vi "Mouse Down Signal.vi"(8 "error in (no error)":errorcluster, 11 "Handle in":refnum<class "Handle.lvclass">) -> (0 "error out":errorcluster, 3 "Handle out":refnum<class "Handle.lvclass">)   [LabVIEW 2021, in "Autocomplete Textbox.lvlib" / "Handle.lvclass"]
uses:
  Handle.lvclass
  ToMain UE.ctl
  ToMain UE action.ctl
  Handle.lvclass/Handle.ctl
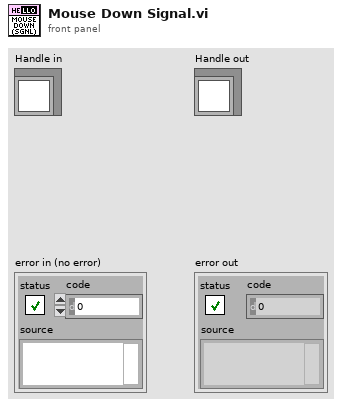
[diagram p1: front panel]
types:
  T1 = typedef "Autocomplete Textbox.lvlib/Handle.lvclass/ToMain UE action.ctl" = enum16{"New List", "Shutdown", "New Value", "Mouse Down (signal)"}
  T2 = typedef "Autocomplete Textbox.lvlib/Handle.lvclass/ToMain UE.ctl" = cluster{"Type":T1, "data":variant}
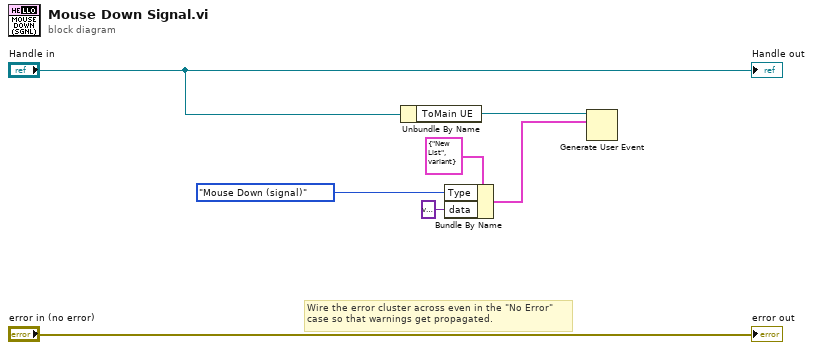
[diagram p0: block diagram]
diagram:
  # "Wire the error cluster across even in the \"No Error\"\ncase so that warnings get propagated."
  n1 = Unbundle By Name("Handle in") -> ("ToMain UE"=w6:refnum<user-event>)
  n2 = Bundle By Name(cluster=T2 {"Type"=enum."New List", "data"=variant} ("event data"), "Type"=ToMain_UE_action."Mouse Down (signal)", "data"=variant) -> (w2:T2)
  n3 = Generate User Event(user event=w6, event data cluster=w2) -> ()  [unwired: 2 in, 2 out]
  "error out" <- "error in (no error)"
  "Handle out" <- "Handle in"
